vi "Distance From Target.vi"(1 "Target Angle (Deg)":dbl, 2 "Camera Angle (Deg)":dbl, 3 "Camera Height (in)":dbl, 4 "Target Height (in)":dbl) -> (0 "Distance (in)":dbl)   [LabVIEW 2019]
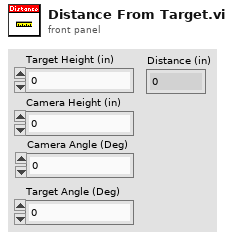
[diagram p1: front panel]
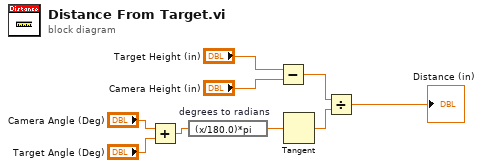
[diagram p0: block diagram]
diagram:
  n1 = Add(x="Camera Angle (Deg)", y="Target Angle (Deg)") -> (x+y=w4:dbl)
  n2 = expression code="(x/180.0)*pi" "degrees to radians"(w4) -> (w3:dbl)
  n3 = Subtract(x="Target Height (in)", y="Camera Height (in)") -> (x-y=w9:dbl)
  n4 = Tangent(1:w3) -> (0:w8:dbl)
  n5 = Divide(x=w9, y=w8) -> (x/y=→"Distance (in)":dbl)
